vi "Initialise 2x2 Array.vi"(9 "element":dbl=1.0, 11 "new diagonal/fill element":dbl=nan) -> (2 "Output Array":dbl[][](array[numeric]))   [LabVIEW 2022 SP3]
uses:
  <vilib>/Analysis/Matrix/Numeric/Conversions/Matrix To Array - RM.vi
  <vilib>/Analysis/Matrix/NI_Matrix.lvlib
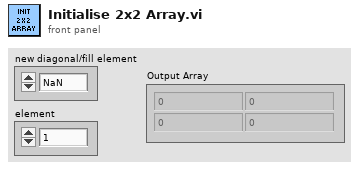
[diagram p1: front panel]
types:
  T1 = typedef "NI_Matrix.lvlib/RealMatrix.ctl" = dbl[][]
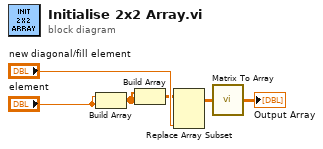
[diagram p0: block diagram]
diagram:
  n1 = Build Array("element", "element") -> (w2:dbl[])
  n2 = Build Array(w2, w2) -> (w4:T1)
  n3 = Replace Array Subset(array=w4, new element="new diagonal/fill element") -> (w6:T1)  [unwired: 2 in]
  n4 = call-poly <vilib>:"Matrix To Array.vi"("Real Matrix"=w6) -> ("Real 2D Array"=→"Output Array":dbl[][])
